vi "Build Dependent Hierarchy Generator.vi"(0 "Build Analyzer in":refnum<class "Build Analyzer.lvclass">, 11 "error in (no error)":errorcluster) -> (4 "dup Build Analyze":refnum<class "Build Analyzer.lvclass">, 6 "Bubbe Up Working Set":refnum<data-value>, 15 "error out":errorcluster)   [LabVIEW 2017, in "CL_G3_VIComponentBuilder.lvlib" / "Build Analyzer.lvclass"]
doc: "Generates the a hierarchy of exports where each node in the hierarchy has as its child nodes the exports that DEPEND on it."
uses:
  Build Analyzer.lvclass
  <userlib>/_Cirrus Logic/LabVIEW Container/Source/Container/Container.lvclass
  Build Analyzer.lvclass/Build Analyzer.ctl
  <userlib>/_Cirrus Logic/LabVIEW Container/Source/Container/Get All Children.vi
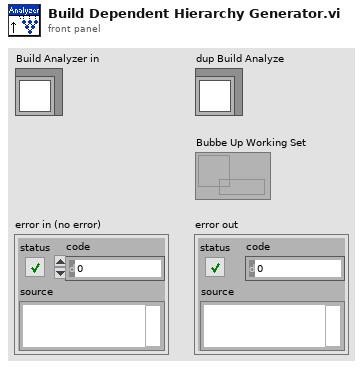
[diagram p1: front panel]
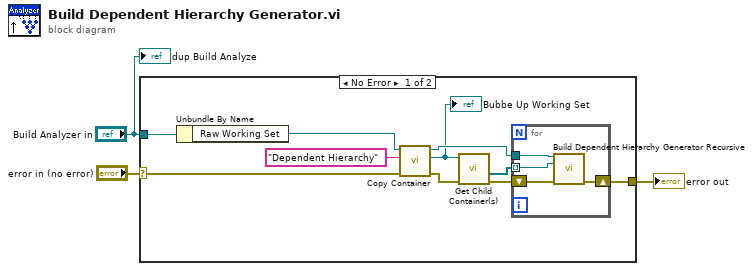
[diagram p0: block diagram]
diagram:
  n1 = case shown="No Error" "error in (no error)" {
    selector: "error in (no error)" -> [w5 w18]
    tunnel: "Build Analyzer in" -> [w9 _]
    tunnel: [w13 w18] -> w2
    frame No Error {
      n2 = Unbundle By Name(w9) -> ("Raw Working Set"=w10:refnum<data-value>)
      n3 = call <userlib>:"Copy Container.vi"("error in (no error)"=w5, "New Container Name"="Dependent Hierarchy" ("Container Name"), "Container"=w10) -> ("error out"=w7:errorcluster, "New Container"=w4:refnum<data-value>, "dup Container"=w12:refnum<data-value>)  [unwired: 6 in]
      "Bubbe Up Working Set" <- w4
      n4 = call-poly <userlib>:"Get Child Container(s).vi"("error in (no error)"=w7, "Container"=w4) -> ("error out"=w6:errorcluster, "Child Containers"=w8:refnum<data-value>[])  [unwired: 6 in, 2 out]
      n5 = for {
        tunnel: w12 -> [w16]
        tunnel: w8 -> [w14] mode=indexing
        shift-right: [w17] -> w13
        shift-left: w6 -> [w15]
        n6 = call "Build Dependent Hierarchy Generator Recursive.vi"("Working Set"=w16, "Next Root"=w14, "error in (no error)"=w15) -> ("error out"=w17:errorcluster)  [unwired: 12 in]
      }
    }
    frame Error {
    }
  }
  "error out" <- w2
  "dup Build Analyze" <- "Build Analyzer in"
